vi "Wait For AT cmd Ready.vi"(7 "After delay (0 msecs)":u32, 8 "error in (no error)":errorcluster, 9 "Timeout (mSecs)":dbl=3000.0, 10 "Initial delay (0 msecs)":u32, 11 "VISA Refnum in":refnum<visa-resource-name>="COM30") -> (0 "error out":errorcluster, 1 "timeout":bool, 2 "Elapsed seconds":dbl format="%#.0f", 3 "VISA Refnum out":refnum<visa-resource-name>="COM99")   [LabVIEW 2013]
uses:
  Test Globals/Global 1.vi
panel:
  out "Com port buffer":string
  # "Waiting for skywire to be \nAT CMD Ready"
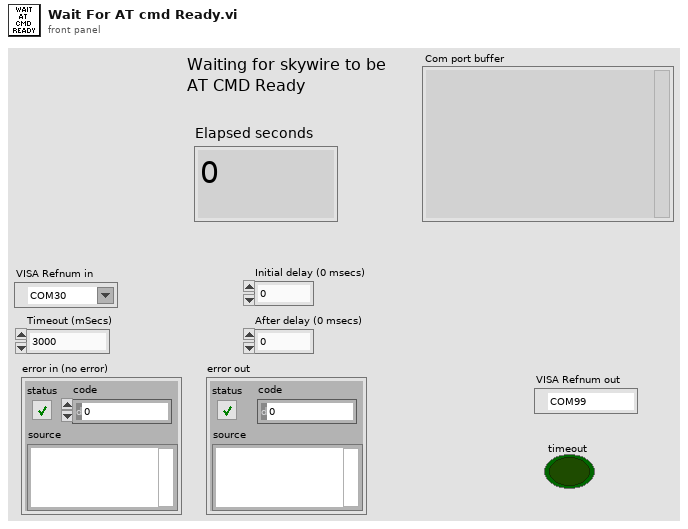
[diagram p1: front panel]
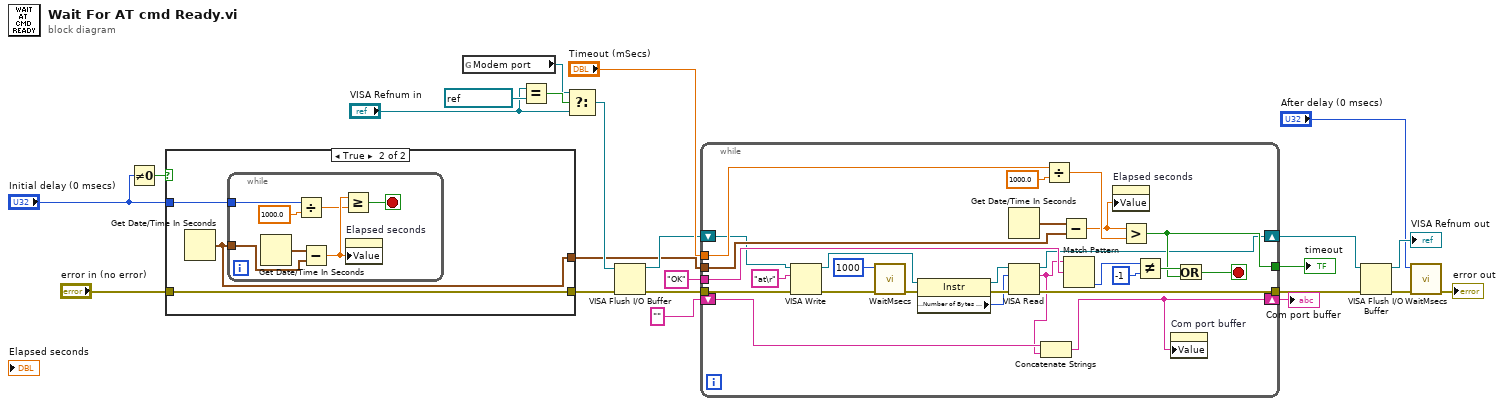
[diagram p0: block diagram]
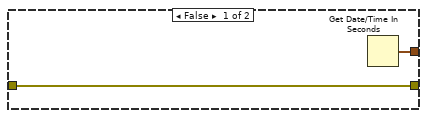
[diagram p2: hidden frame]
diagram:
  n1 = Not Equal To 0?(x="Initial delay (0 msecs)") -> (x != 0?=w7:bool)
  n2 = case shown="True" w7 {
    tunnel: "Initial delay (0 msecs)" -> [_ w28]
    tunnel: [w25 w27] -> w4
    tunnel: "error in (no error)" -> [w25 w27]
    tunnel: [w24 w26] -> w3
    frame False {
      n3 = Get Date/Time In Seconds() -> (seconds since 1Jan1904=w24:timestamp)
    }
    frame True {
      n4 = Get Date/Time In Seconds() -> (seconds since 1Jan1904=w26:timestamp)
      n5 = while {
        tunnel: w26 -> [w32]
        tunnel: w28 -> [w31]
        stop <- w30 stop-if-true
        n6 = Get Date/Time In Seconds() -> (seconds since 1Jan1904=w29:timestamp)
        n7 = Divide(x=w31, y=1000.0) -> (x/y=w33:dbl)
        n8 = Subtract(x=w29, y=w32) -> (x-y=w35:dbl)
        n9 = Greater Or Equal?(x=w35, y=w33) -> (x >= y?=w30:bool)
        n10 = property on="Elapsed seconds" class="DigNum (strict)"("Value"=w35) -> ()  [unwired: 2 in, 2 out]
      }
    }
  }
  n11 = global read "Global 1.vi" "Modem port"() -> (w13:refnum<visa-resource-name>)
  n12 = Equal?(x="VISA Refnum in", y=refnum<visa-resource-name> "COM99" ("VISA Refnum in")) -> (x = y?=w14:bool)
  n13 = Select(t=w13, s=w14, f="VISA Refnum in") -> (s? t:f=w11:refnum<visa-resource-name>)
  n14 = VISA Flush I/O Buffer(VISA resource name=w11, error in (no error)=w4) -> (VISA resource name out=w19:refnum<visa-resource-name>, error out=w20:errorcluster)  [unwired: 1 in]
  n15 = while {
    tunnel: w20 -> [w48]
    tunnel: "OK" ("Wait for") -> [w57]
    tunnel: [w40] -> w17
    tunnel: [w51] -> w22
    tunnel: "Timeout (mSecs)" -> [w56]
    tunnel: w3 -> [w53]
    shift-right: [w49] -> w18
    shift-left: w19 -> [w44]
    shift-right: [w36] -> w1
    shift-left: "" -> [w38]
    stop <- w42 stop-if-true
    n16 = VISA Write(VISA resource name=w44, write buffer="at\r", error in (no error)=w48) -> (VISA resource name out=w43:refnum<visa-resource-name>, error out=w47:errorcluster)  [unwired: 1 out]
    n17 = call "WaitMsecs.vi"("error in (no error)"=w47, "Wait Msecs"=u32 1000) -> ("error out"=w45:errorcluster)  [unwired: 9 in]
    n18 = property class="Instr"(reference=w43, error in=w45) -> (reference out=w60:refnum<visa-resource-name>, error out=w62:errorcluster, "Serial Settings:Number of Bytes at Serial Port"=w61:u32)
    n19 = Get Date/Time In Seconds() -> (seconds since 1Jan1904=w54:timestamp)
    n20 = VISA Read(VISA resource name=w60, byte count=w61, error in (no error)=w62) -> (VISA resource name out=w49:refnum<visa-resource-name>, read buffer=w37:string, error out=w40:errorcluster)  [unwired: 1 out]
    n21 = Concatenate Strings(w38, w37) -> (w36:string)
    n22 = Divide(x=w56, y=1000.0) -> (x/y=w52:dbl)
    n23 = Subtract(x=w54, y=w53) -> (x-y=w39:dbl)
    n24 = Match Pattern(string=w37, regular expression=w57) -> (offset past match=w59:i32)  [unwired: 1 in, 3 out]
    n25 = property on="Elapsed seconds" class="DigNum (strict)"("Value"=w39) -> ()  [unwired: 2 in, 2 out]
    n26 = Greater?(x=w39, y=w52) -> (0:w51:bool)
    n27 = Not Equal?(x=w59, y=-1) -> (x != y?=w55:bool)
    n28 = property on="Com port buffer" class="Str"("Value"=w36) -> ()  [unwired: 2 in, 2 out]
    n29 = Or(x=w55, y=w51) -> (x .or. y?=w42:bool)
  }
  "timeout" <- w22
  "Com port buffer" <- w1
  n30 = VISA Flush I/O Buffer(VISA resource name=w18, error in (no error)=w17) -> (VISA resource name out=→"VISA Refnum out":refnum<visa-resource-name>, error out=w10:errorcluster)  [unwired: 1 in]
  n31 = call "WaitMsecs.vi"("error in (no error)"=w10, "Wait Msecs"="After delay (0 msecs)") -> ("error out"=→"error out":errorcluster)  [unwired: 9 in]
